vi "XNET Database Merge (Frame).vi"(0 "target cluster in":refnum<k21>, 1 "wait for complete? (T)":bool=TRUE, 5 "source frame":refnum<k21>, 7 "copy mode":T1 items=["Copy using source", "Copy using destination", "Merge using source", "Merge using destination"], 9 "prefix":string, 11 "error in (no error)":errorcluster) -> (3 "percent complete":u32, 4 "target cluster out":refnum<k21>, 15 "error out":errorcluster)   [LabVIEW 2018]
doc: "Adds the source frame to the target cluster."
uses:
  XNET Merge Copy Mode.ctl
  nixlvapi.dll
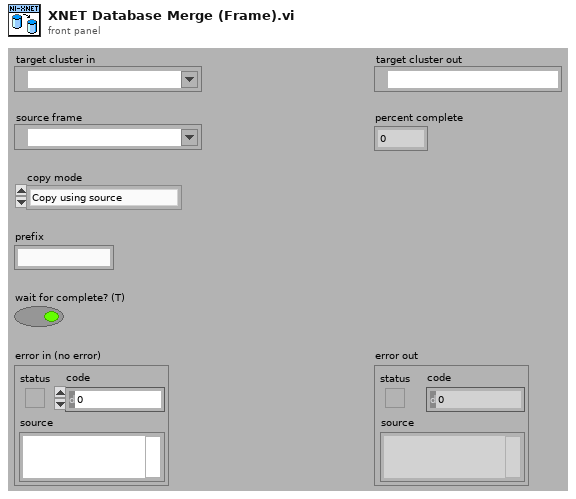
[diagram p1: front panel]
types:
  T1 = typedef "XNET Merge Copy Mode.ctl" = u32
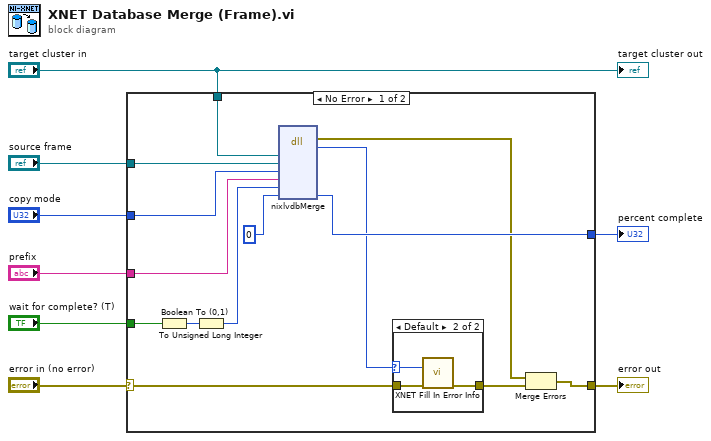
[diagram p0: block diagram]
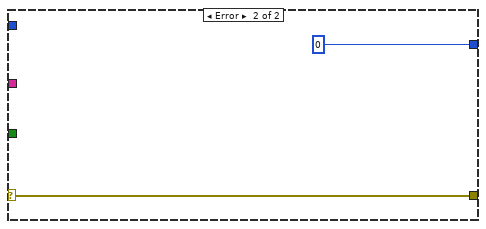
[diagram p3: hidden frame]
diagram:
  n1 = case shown="No Error" "error in (no error)" {
    selector: "error in (no error)" -> [w13 w28]
    tunnel: "target cluster in" -> [w22 _]
    tunnel: "source frame" -> [w21 _]
    tunnel: "copy mode" -> [w20 _]
    tunnel: "prefix" -> [w19 _]
    tunnel: "wait for complete? (T)" -> [w17 _]
    tunnel: [w14 u32 0 ("PercentComplete")] -> w3
    tunnel: [w10 w28] -> w1
    frame No Error {
      n2 = Boolean To (0,1)(Boolean=w17) -> (0, 1=w18:i16)
      n3 = To Unsigned Long Integer(number=w18) -> (unsigned 32bit integer=w16:u32)
      n4 = dll-call lib="nixlvapi.*" fn="nixlvdbMerge"("TargetClusterRef"=w22, "SourceObjRef"=w21, "CopyMode"=w20, "Prefix"=w19, "WaitForComplete"=w16, "PercentComplete"=u32 0) -> (error out=w9:errorcluster, "return type"=w12:i32, "PercentComplete"=w14:u32)  [unwired: 8 in, 1 out]
      n5 = case shown="Default" w12 {
        selector: w12 -> [_ w24]
        tunnel: w13 -> [w23 w26]
        tunnel: [w23 w25] -> w11
        frame 0 {
        }
        frame Default {
          n6 = call "XNET Fill In Error Info.vi"("status code"=w24, "error in"=w26) -> ("error out"=w25:errorcluster)  [unwired: 13 out]
        }
      }
      n7 = Merge Errors(w9, w11) -> (w10:errorcluster)
    }
    frame Error {
    }
  }
  "percent complete" <- w3
  "error out" <- w1
  "target cluster out" <- "target cluster in"
